vi "Clear Queue.vi"(8 "error in (no error)":errorcluster) -> (0 "error out":errorcluster, 2 "remaining elements":T1[](array[typedef]))   [LabVIEW 2020, in "Controller.lvlib"]
uses:
  Controller.lvlib
  Private Controls/Element.ctl
  Private Controls/Module Action.ctl
  Queue FGV Action.ctl
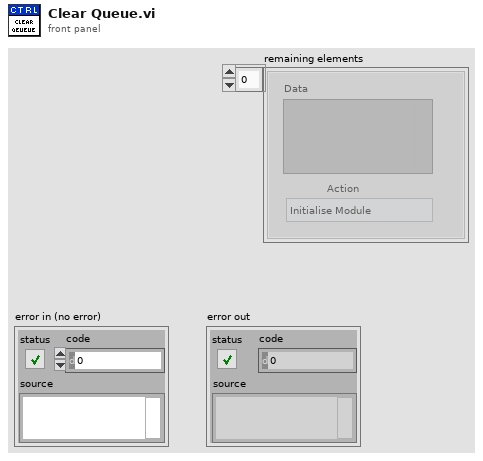
[diagram p1: front panel]
types:
  T1 = typedef "Controller.lvlib/Element.ctl" = cluster{"Action":T2, "Data":variant}
  T2 = typedef "Controller.lvlib/Module Action.ctl" = enum16{"Initialise Module", "Connect", "Setup", "Pause", "Start", "Search Network", "Get Local", "Process Results", "Stop", "Show Match", "Show Full", "Get UI Refs", "Wait: Time Elapsed", "Error", "Exit"}
  T3 = typedef "Controller.lvlib/Queue FGV Action.ctl" = enum16{"Get", "Set", "Release"}
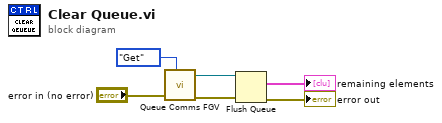
[diagram p0: block diagram]
diagram:
  n1 = call "Queue Comms FGV.vi"("Action"=Queue_FGV_Action."Get", "error in (no error)"="error in (no error)") -> ("error out"=w4:errorcluster, "queue In"=w3:refnum<queue>)  [unwired: 8 in]
  n2 = Flush Queue(queue=w3, error in (no error)=w4) -> (remaining elements=→"remaining elements":T1[], error out=→"error out":errorcluster)  [unwired: 1 out]
